vi "DEBUG-修改窗格最小大小-直接复制粘贴到VI中去.vi"() -> ()   [LabVIEW 2013]
uses:
  <vilib>/Utility/miscctls.llb/LVPoint32TypeDef.ctl
  <vilib>/Utility/miscctls.llb/LVPointTypeDef.ctl
  <vilib>/Utility/miscctls.llb/LVBoundsTypeDef.ctl
panel:
  out "坐标":T1
  out "经过窗口最小窗格大小":T2
  out "经过窗口边界":T3 caption="边界"
  out "经过窗口":string
  out "窗格引用":refnum<vi>
  out "选中窗格":string
  out "停止DEBUG":bool=TRUE
  in  "选中窗口最小窗格大小 2":T2 caption="经过窗口最小窗格大小"
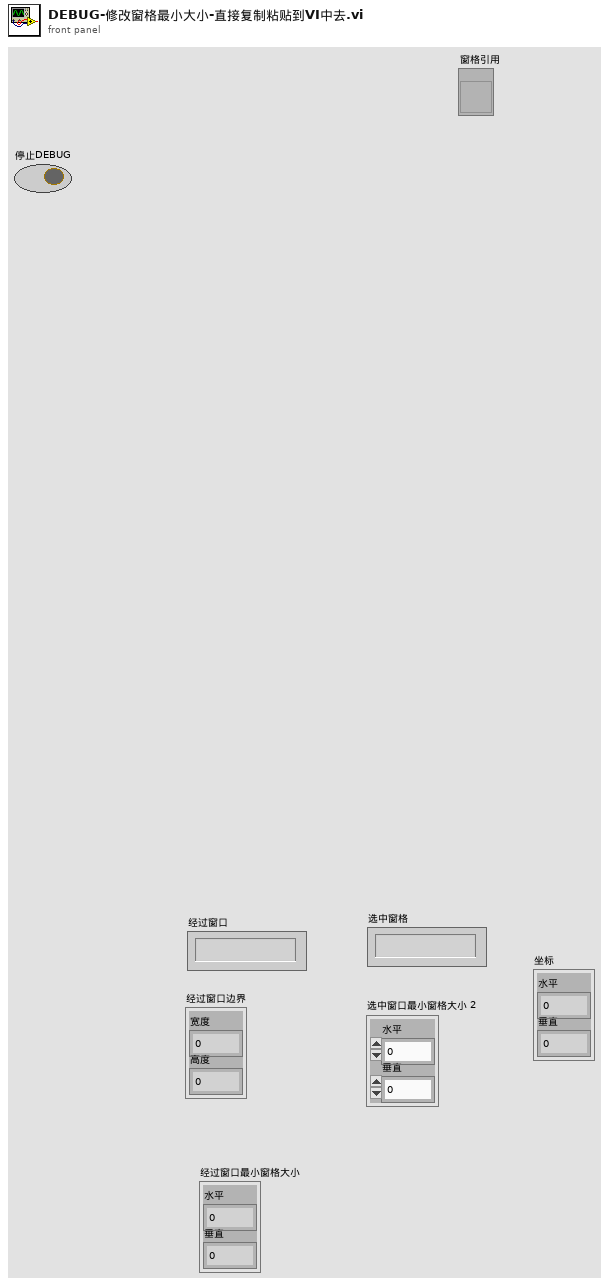
[diagram p1: front panel]
types:
  T1 = typedef "LVPoint32TypeDef.ctl" = cluster{"Horizontal":i32, "Vertical":i32}
  T2 = typedef "LVPointTypeDef.ctl" = cluster{"Horizontal":i16, "Vertical":i16}
  T3 = typedef "LVBoundsTypeDef.ctl" = cluster{"Width":u32, "Height":u32}
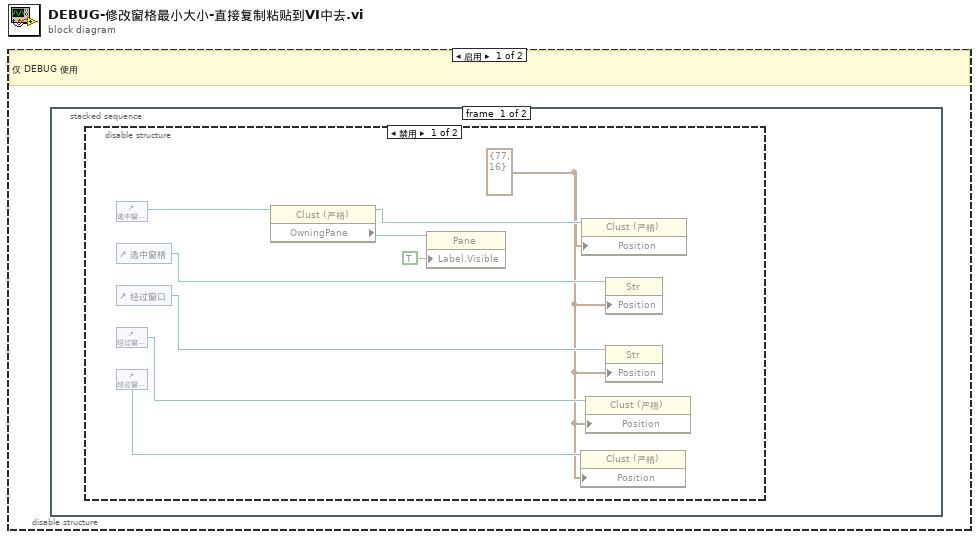
[diagram p0: block diagram]
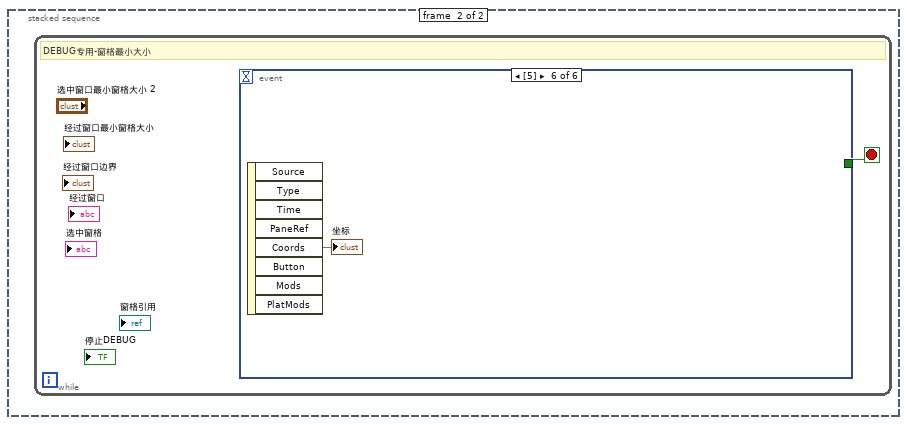
[diagram p3: hidden frame]
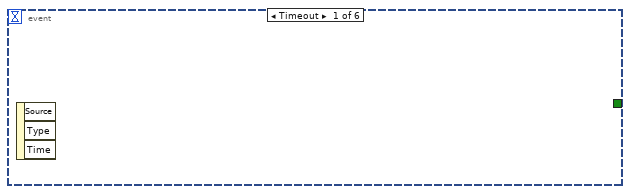
[diagram p4: hidden frame]
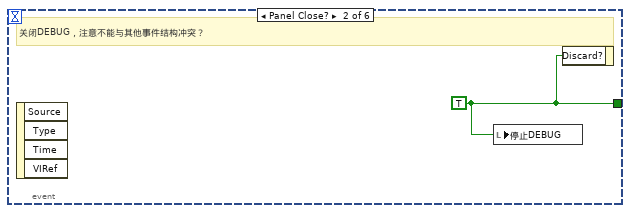
[diagram p5: hidden frame]
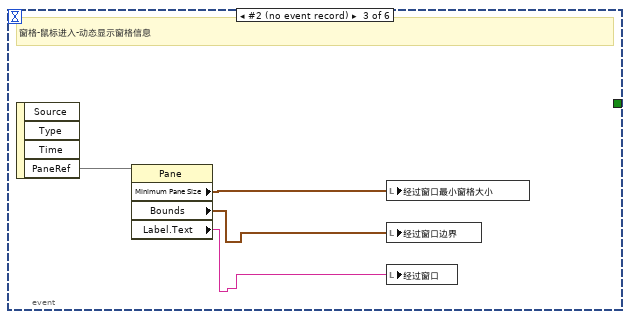
[diagram p6: hidden frame]
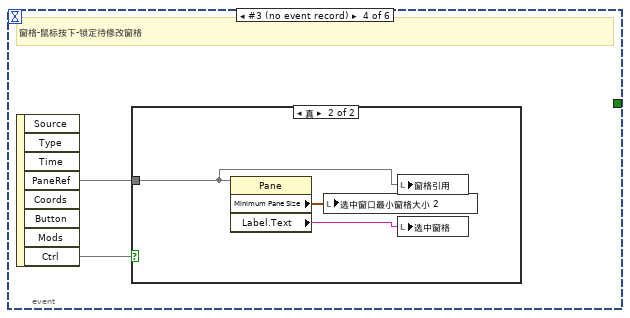
[diagram p7: hidden frame]
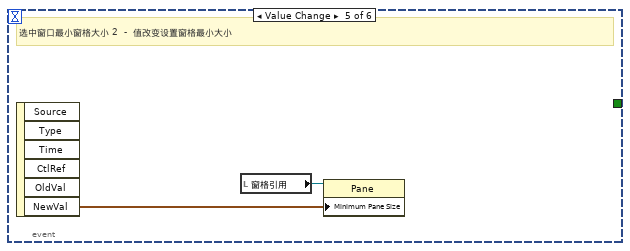
[diagram p9: hidden frame]
diagram:
  n1 = disable-structure shown="启用" {
    frame Enabled {
      # "仅 DEBUG 使用"
      n2 = stacked-sequence {
        frame #0 {
          n3 = disable-structure shown="禁用" {
            frame Disabled {
              w1 = T1 {"Horizontal"=77, "Vertical"=16} ("坐标")
              n4 = control-ref of="选中窗口最小窗格大小 2"() -> (w9:refnum<vi>)
              n5 = control-ref of="选中窗格"() -> (w5:refnum<vi>)
              n6 = control-ref of="经过窗口"() -> (w4:refnum<vi>)
              n7 = control-ref of="经过窗口边界"() -> (w3:refnum<vi>)
              n8 = control-ref of="经过窗口最小窗格大小"() -> (w2:refnum<vi>)
              n9 = property class="Clust (严格)"(reference=w9) -> (reference out=w6:refnum<vi>, "OwningPane"=w8:refnum<vi>)  [unwired: 1 in, 1 out]
              n10 = property class="Pane"(reference=w8, "Label.Visible"=TRUE ("标签.可见")) -> ()  [unwired: 1 in, 2 out]
              n11 = property class="Clust (严格)"(reference=w2, "Position"=w1) -> ()  [unwired: 1 in, 2 out]
              n12 = property class="Clust (严格)"(reference=w6, "Position"=w1) -> ()  [unwired: 1 in, 2 out]
              n13 = property class="Clust (严格)"(reference=w3, "Position"=w1) -> ()  [unwired: 1 in, 2 out]
              n14 = property class="Str"(reference=w5, "Position"=w1) -> ()  [unwired: 1 in, 2 out]
              n15 = property class="Str"(reference=w4, "Position"=w1) -> ()  [unwired: 1 in, 2 out]
            }
            frame Enabled {
            }
          }
        }
        frame #1 {
          n16 = while {
            stop <- w10 stop-if-true
            # "DEBUG专用-窗格最小大小"
            n17 = event shown="[5]" {
              selector: _ -> [_ _ _ _ _ _]
              dyn-events: _ -> [_ _ _ _ _ _]
              timeout: _ -> [_ _ _ _ _ _]
              tunnel: [_ w11 _ _ _ _] -> w10
              event Timeout {
                n18 = event-data() -> ()  [unwired: 1 in, 3 out]
              }
              event Panel Close? {
                w11 = TRUE ("放弃？")
                # "关闭DEBUG，注意不能与其他事件结构冲突？"
                n19 = event-data() -> ()  [unwired: 1 in, 4 out]
                n20 = local write "停止DEBUG"(w11) -> ()
                n21 = event-data("Discard?"=w11) -> ()  [unwired: 1 in, 1 out]
              }
              event #2 (no event record) {
                # "窗格-鼠标进入-动态显示窗格信息"
                n22 = event-data() -> ("PaneRef"=w15)  [unwired: 1 in, 3 out]
                n23 = property class="Pane"(reference=w15) -> ("Minimum Pane Size"=w14:T2, "Bounds"=w13:T3, "Label.Text"=w12:string)  [unwired: 1 in, 2 out]
                n24 = local write "经过窗口最小窗格大小"(w14) -> ()
                n25 = local write "经过窗口边界"(w13) -> ()
                n26 = local write "经过窗口"(w12) -> ()
              }
              event #3 (no event record) {
                # "窗格-鼠标按下-锁定待修改窗格"
                n27 = event-data() -> ("PaneRef"=w17, "Ctrl"=w16)  [unwired: 1 in, 6 out]
                n28 = case shown="真" w16 {
                  tunnel: w17 -> [_ w19]
                  frame False {
                  }
                  frame True {
                    n29 = property class="Pane"(reference=w19) -> ("Minimum Pane Size"=w20:T2, "Label.Text"=w18:string)  [unwired: 1 in, 2 out]
                    n30 = local write "选中窗口最小窗格大小 2"(w20) -> ()
                    n31 = local write "窗格引用"(w19) -> ()
                    n32 = local write "选中窗格"(w18) -> ()
                  }
                }
              }
              event Value Change {
                # "选中窗口最小窗格大小 2  -  值改变设置窗格最小大小"
                n33 = event-data() -> ("NewVal"=w21:T2)  [unwired: 1 in, 5 out]
                n34 = local read "窗格引用"() -> (w22:refnum<vi>)
                n35 = property class="Pane"(reference=w22, "Minimum Pane Size"=w21) -> ()  [unwired: 1 in, 2 out]
              }
              event #5 (no event record) {
                n36 = event-data() -> ("Coords"=→"坐标")  [unwired: 1 in, 7 out]
              }
            }
          }
        }
      }
    }
    frame Disabled {
    }
  }
